vi "sequential on_off - fluigent.vi"() -> ()   [LabVIEW 2018]
doc: "Manually blink and LED attached to a digital output channel of a LINX device by clicking and LED control in LabVIEW."
uses:
  <userlib>/Fluigent/Fluigent MFCS/FluigentMFCS_Full.llb/MFCS_EZ Detect.vi
  <userlib>/Fluigent/Fluigent MFCS/FluigentMFCS_Full.llb/MFCS_EZ Initialization.vi
  <userlib>/Fluigent/Fluigent MFCS/FluigentMFCS_Full.llb/MFCS_EZ Read All Channels Pressure.vi
  <userlib>/Fluigent/Fluigent MFCS/FluigentMFCS_Full.llb/MFCS_EZ Write Channel Pressure.vi
  <userlib>/Fluigent/Fluigent MFCS/FluigentMFCS_Full.llb/MFCS_EZ Close.vi
panel:
  in  "Alpha_8":dbl
  in  "Alpha_7":dbl
  in  "Alpha_6":dbl
  in  "Alpha_5":dbl
  in  "Alpha_4":dbl
  in  "Alpha_3":dbl
  in  "Alpha_2":dbl
  in  "Alpha_1":dbl
  in  "Delay_outlet(ms)":dbl
  in  "Delay_inlet(ms)":dbl
  out "All Channels Pressure":dbl[](array[numeric])
  in  "ch_4_LOW 2":dbl
  in  "ch_3_LOW 2":dbl
  in  "ch_2_LOW 2":dbl
  in  "ch_1_LOW 2":dbl
  in  "ch_4_HIGH 2":dbl
  in  "ch_3_HIGH 2":dbl
  in  "ch_2_HIGH 2":dbl
  in  "ch_1_HIGH 2":dbl
  in  "valve_8_pressure":dbl
  in  "valve_7_pressure":dbl
  in  "valve_6_pressure":dbl
  in  "valve_5_pressure":dbl
  in  "valve_4_pressure":dbl
  in  "valve_3_pressure":dbl
  in  "valve_2_pressure":dbl
  in  "valve_1_pressure":dbl
  in  "ch_4_LOW":dbl
  in  "ch_4_HIGH":dbl
  in  "ch_3_LOW":dbl
  in  "ch_3_HIGH":dbl
  in  "ch_2_LOW":dbl
  in  "ch_2_HIGH":dbl
  in  "ch_1_LOW":dbl
  in  "ch_1_HIGH":dbl
  in  "Chnl_1":bool
  in  "Chnl_2":bool
  in  "Chnl_4":bool
  in  "Chnl_3":bool
  in  "Delay (ms)":dbl
  in  "Mode Selection":enum32{"Manual Control", "Sequential Control"}(radio)
  out "ch_4":bool
  out "ch_3":bool
  out "ch_2":bool
  out "ch_1":bool
  out "id_8":bool
  out "id_7":bool
  out "id_6":bool
  out "id_5":bool
  out "id_4":bool
  out "id_3":bool
  out "id_2":bool
  out "id_1":bool
  in  "stop":bool
  in  "Valve 8":bool
  in  "Valve 7":bool
  in  "Valve 6":bool
  in  "Valve 5":bool
  in  "Valve 4":bool
  in  "Valve 3":bool
  in  "Valve 2":bool
  in  "Valve_1":bool
  # "Manual Control:"
  # "LINX Device Settings"
  # "Sequential Control:"
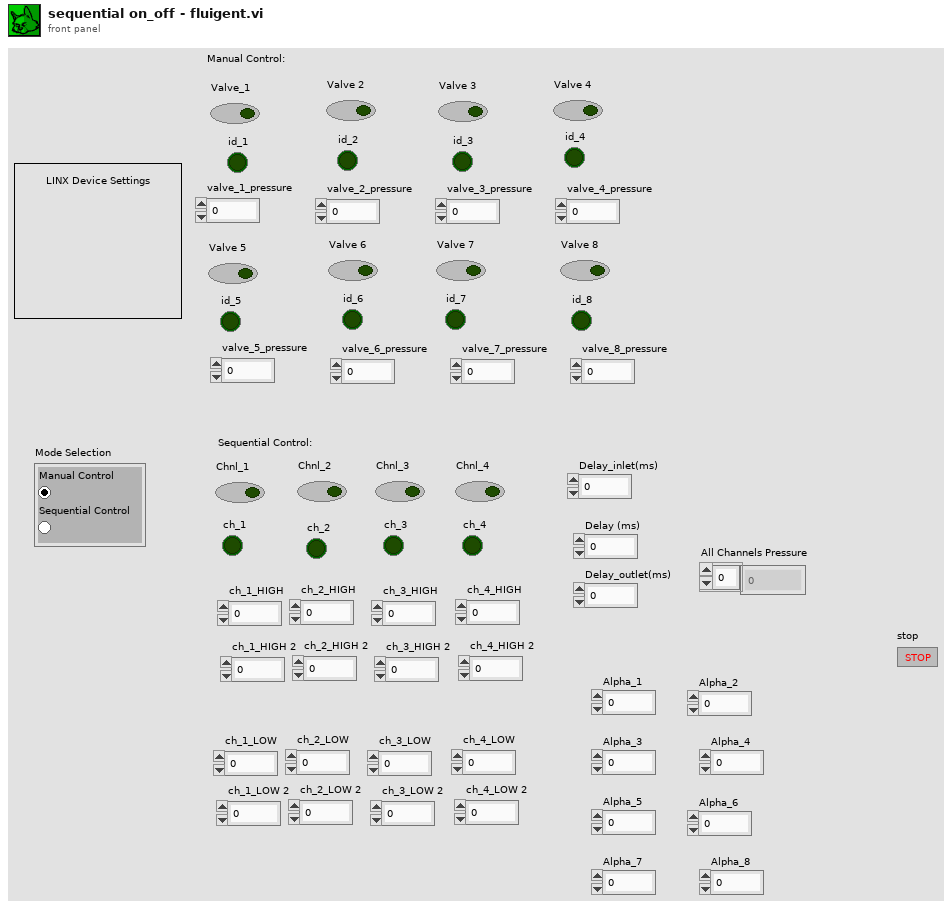
[diagram p1: front panel]
types:
  T1 = typedef "_EZmfcsSN.ctl" = u16
  T2 = typedef "_mfcs_EZ_handle.ctl" = u64
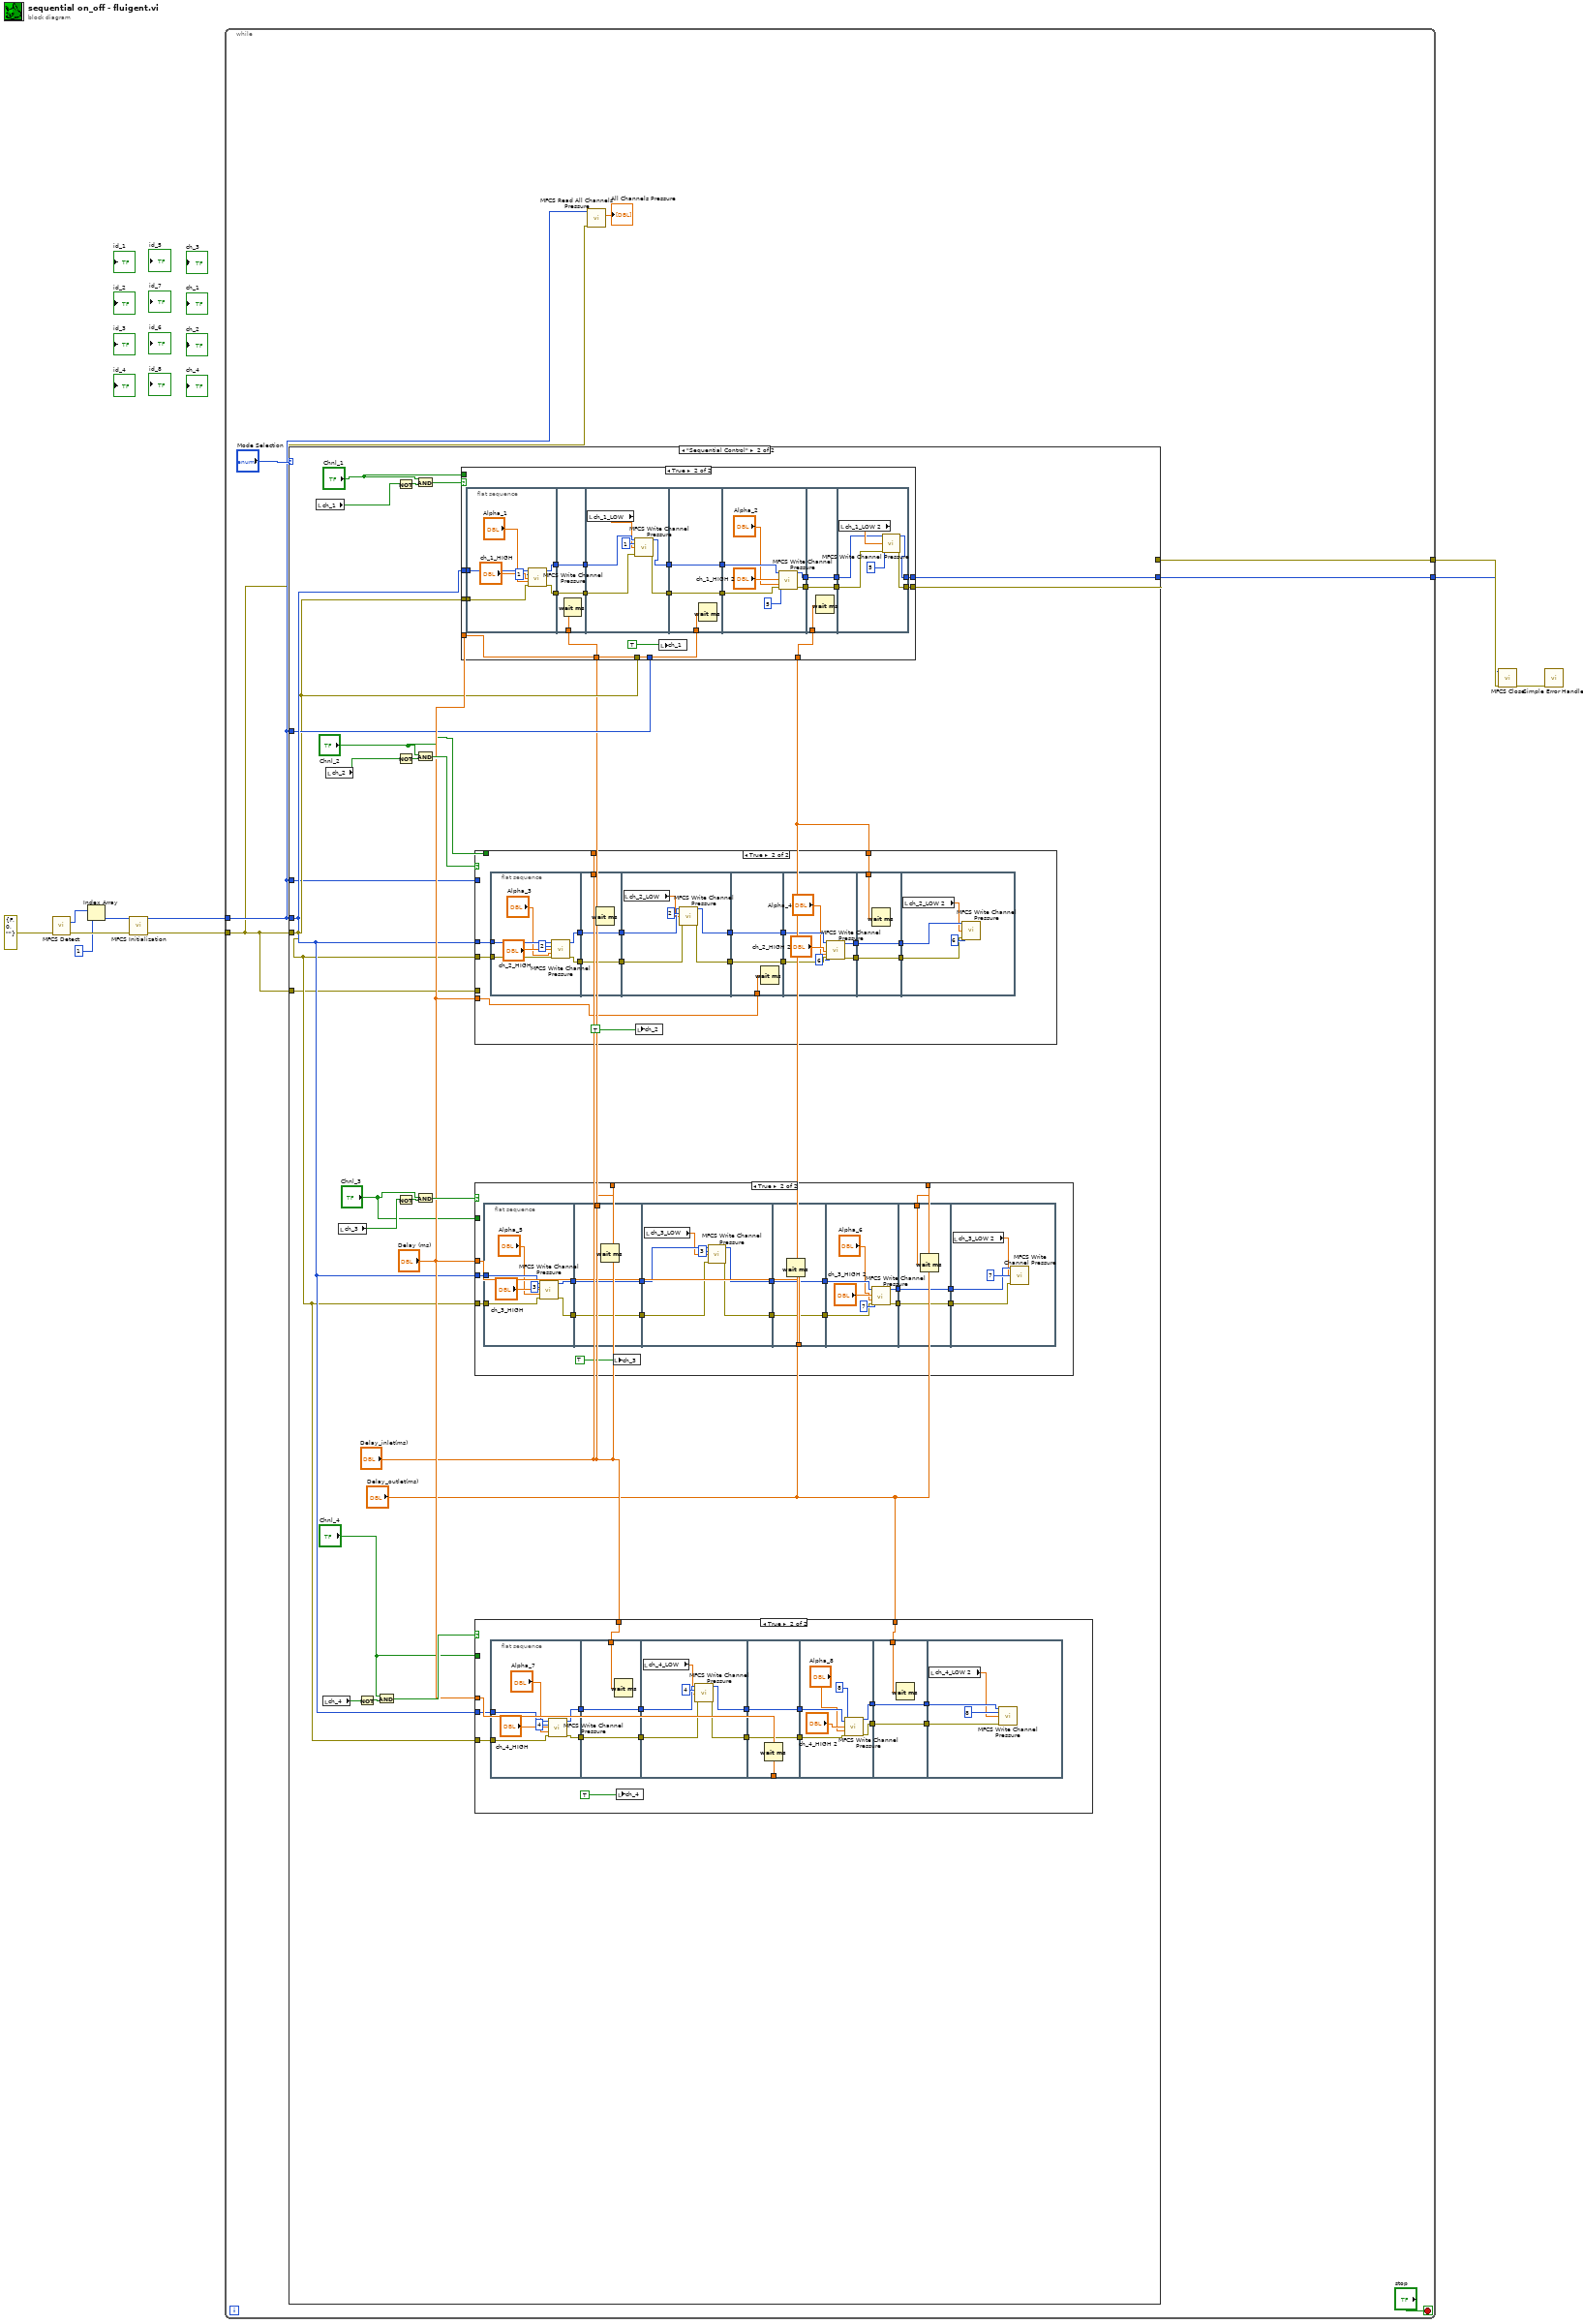
[diagram p0: block diagram]
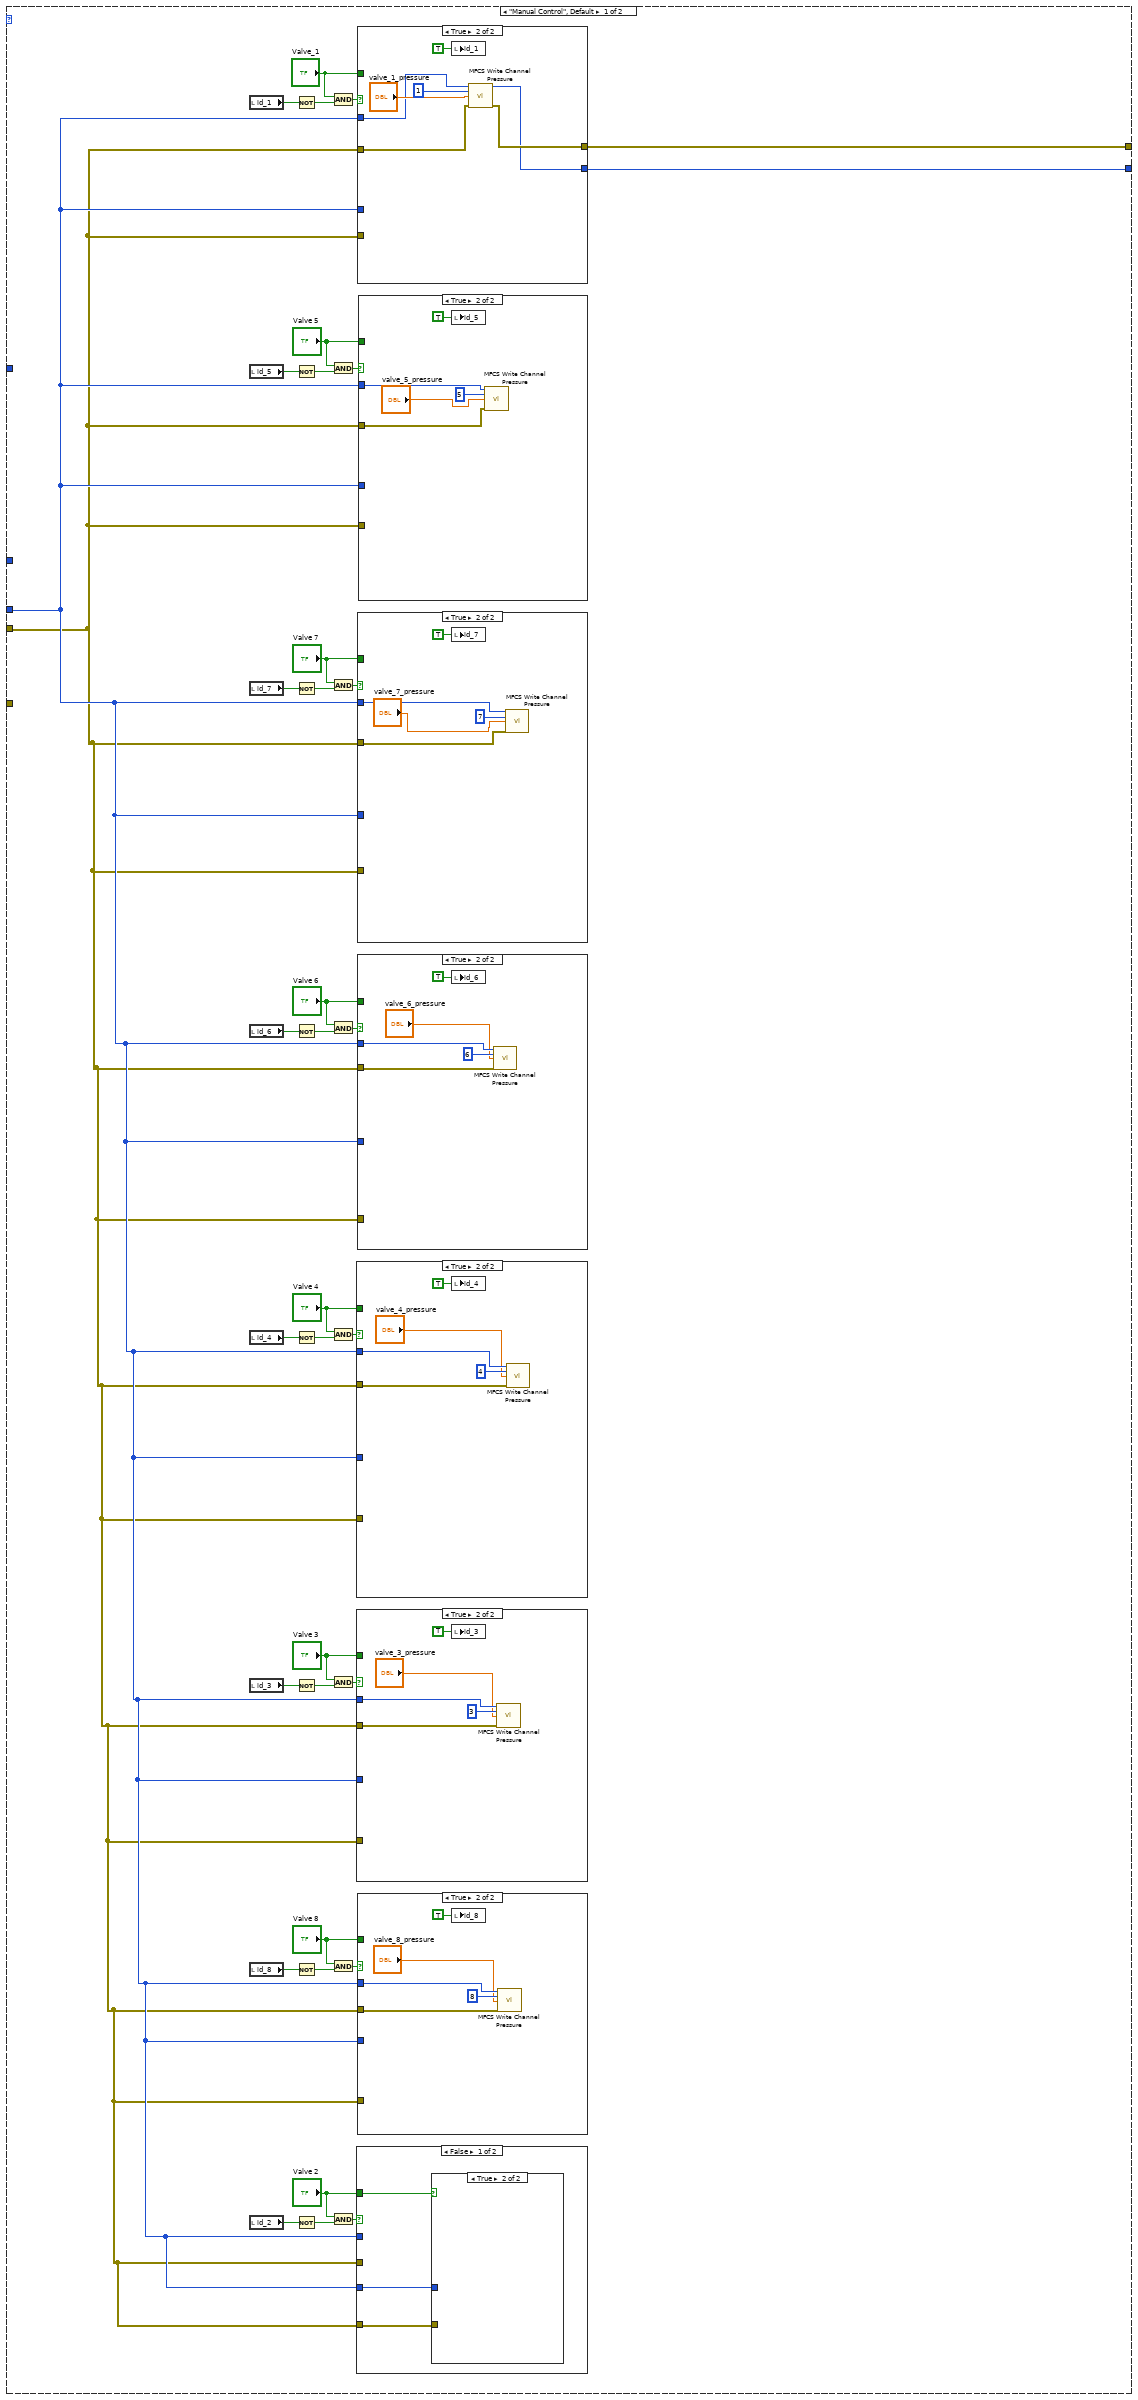
[diagram p2: hidden frame]
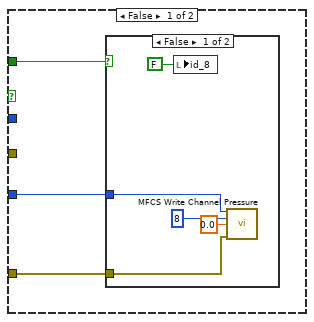
[diagram p3: hidden frame]
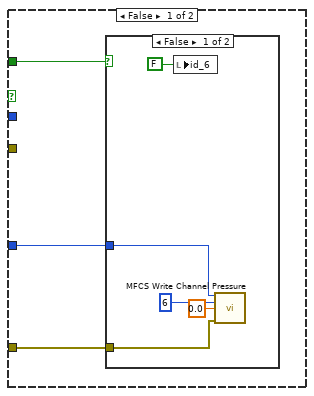
[diagram p5: hidden frame]
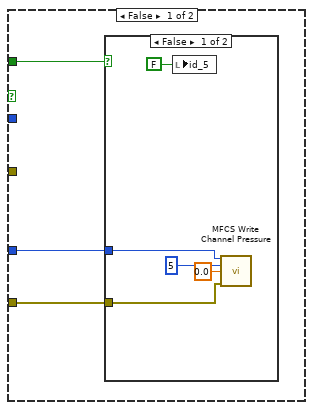
[diagram p7: hidden frame]
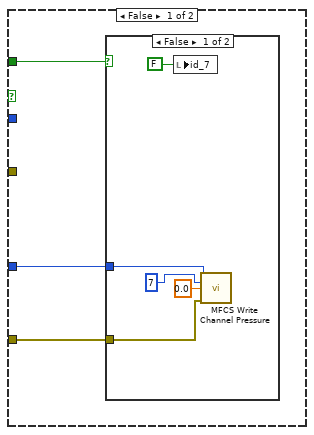
[diagram p9: hidden frame]
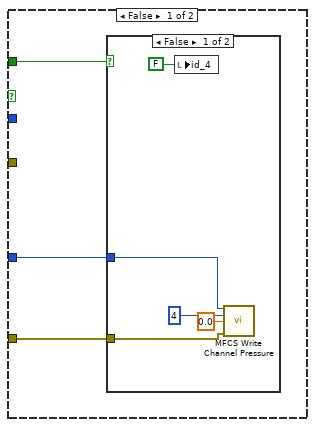
[diagram p11: hidden frame]
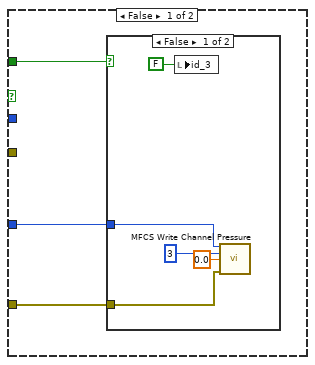
[diagram p13: hidden frame]
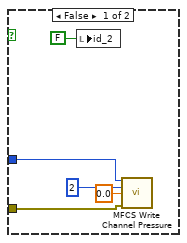
[diagram p15: hidden frame]
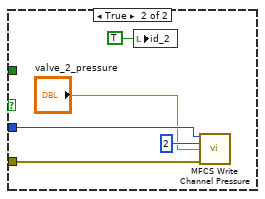
[diagram p16: hidden frame]
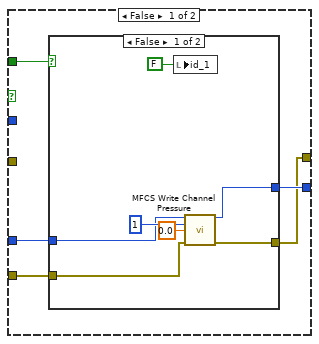
[diagram p17: hidden frame]
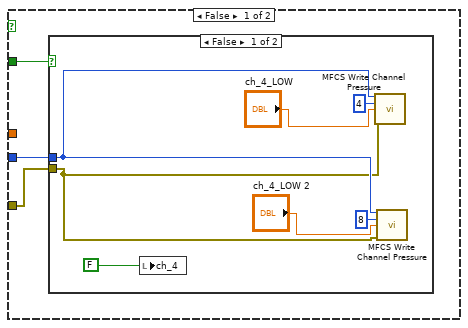
[diagram p19: hidden frame]
diagram:
  n1 = call-poly <userlib>:"MFCS Detect.vi"("error in (no error)"=errorcluster {"status"=FALSE, "code"=0, "source"=""}) -> ("[SN MFCS_EZ]"=w9:T1[], "error out"=w8:errorcluster)  [unwired: 13 in]
  n2 = Index Array(array=w9, index=1) -> (element=w7:T1)
  n3 = call-poly <userlib>:"MFCS Initialization.vi"("SN MFCS_EZ"=w7, "error in (no error)"=w8) -> ("MFCS_EZ_out"=w5:T2, "error out"=w6:errorcluster)  [unwired: 10 in, 2 out]
  n4 = while {
    tunnel: w6 -> [w12]
    tunnel: w5 -> [w13]
    tunnel: [w15] -> w3
    tunnel: [w14] -> w2
    stop <- "stop" stop-if-true
    n5 = case shown="\"Sequential Control\"" "Mode Selection" {
      tunnel: w12 -> [w18 w170]
      tunnel: w13 -> [w19 w172]
      tunnel: [w21 w173] -> w15
      tunnel: [w20 w174] -> w14
      tunnel: w13 -> [_ w171]
      tunnel: w13 -> [_ w169]
      tunnel: w12 -> [_ w168]
      frame "Manual Control", Default {
        n6 = local read "id_1"() -> (w23:bool)
        n7 = local read "id_5"() -> (w36:bool)
        n8 = local read "id_7"() -> (w38:bool)
        n9 = local read "id_6"() -> (w37:bool)
        n10 = local read "id_4"() -> (w35:bool)
        n11 = local read "id_3"() -> (w34:bool)
        n12 = local read "id_8"() -> (w39:bool)
        n13 = local read "id_2"() -> (w27:bool)
        n14 = Not(x=w23) -> (.not. x?=w24:bool)
        n15 = Not(x=w36) -> (.not. x?=w46:bool)
        n16 = Not(x=w38) -> (.not. x?=w42:bool)
        n17 = Not(x=w37) -> (.not. x?=w44:bool)
        n18 = Not(x=w35) -> (.not. x?=w32:bool)
        n19 = Not(x=w34) -> (.not. x?=w29:bool)
        n20 = Not(x=w39) -> (.not. x?=w40:bool)
        n21 = Not(x=w27) -> (.not. x?=w26:bool)
        n22 = And(x="Valve_1", y=w24) -> (x .and. y?=w22:bool)
        n23 = And(x="Valve 5", y=w46) -> (x .and. y?=w47:bool)
        n24 = And(x="Valve 7", y=w42) -> (x .and. y?=w43:bool)
        n25 = And(x="Valve 6", y=w44) -> (x .and. y?=w45:bool)
        n26 = And(x="Valve 4", y=w32) -> (x .and. y?=w33:bool)
        n27 = And(x="Valve 3", y=w29) -> (x .and. y?=w30:bool)
        n28 = And(x="Valve 8", y=w40) -> (x .and. y?=w41:bool)
        n29 = And(x="Valve 2", y=w26) -> (x .and. y?=w25:bool)
        n30 = case shown="True" w33 {
          tunnel: "Valve 4" -> [w108 _]
          tunnel: w19 -> [_ w116]
          tunnel: w18 -> [_ w115]
          tunnel: w19 -> [w107 _]
          tunnel: w18 -> [w106 _]
          frame False {
            n31 = case shown="False" w108 {
              tunnel: w107 -> [w110 _]
              tunnel: w106 -> [w109 _]
              frame False {
                n32 = local write "id_4"(FALSE) -> ()
                n33 = call-poly <userlib>:"MFCS Write Channel Pressure.vi"("MFCS_EZ"=w110, "Channel Number (default=1)"=u8 4, "Pressure (mBar)"=0.0, "error in (no error)"=w109) -> ()  [unwired: 10 in, 2 out]
              }
              frame True {
              }
            }
          }
          frame True {
            n34 = local write "id_4"(TRUE) -> ()
            n35 = call-poly <userlib>:"MFCS Write Channel Pressure.vi"("MFCS_EZ"=w116, "Channel Number (default=1)"=u8 4, "Pressure (mBar)"="valve_4_pressure", "error in (no error)"=w115) -> ()  [unwired: 10 in, 2 out]
          }
        }
        n36 = case shown="True" w30 {
          tunnel: "Valve 3" -> [w121 _]
          tunnel: w19 -> [_ w129]
          tunnel: w18 -> [_ w128]
          tunnel: w19 -> [w120 _]
          tunnel: w18 -> [w119 _]
          frame False {
            n37 = case shown="False" w121 {
              tunnel: w120 -> [w123 _]
              tunnel: w119 -> [w122 _]
              frame False {
                n38 = local write "id_3"(FALSE) -> ()
                n39 = call-poly <userlib>:"MFCS Write Channel Pressure.vi"("MFCS_EZ"=w123, "Channel Number (default=1)"=u8 3, "Pressure (mBar)"=0.0, "error in (no error)"=w122) -> ()  [unwired: 10 in, 2 out]
              }
              frame True {
              }
            }
          }
          frame True {
            n40 = local write "id_3"(TRUE) -> ()
            n41 = call-poly <userlib>:"MFCS Write Channel Pressure.vi"("MFCS_EZ"=w129, "Channel Number (default=1)"=u8 3, "Pressure (mBar)"="valve_3_pressure", "error in (no error)"=w128) -> ()  [unwired: 10 in, 2 out]
          }
        }
        n42 = case shown="False" w25 {
          tunnel: "Valve 2" -> [w134 _]
          tunnel: w19 -> [_ w142]
          tunnel: w18 -> [_ w141]
          tunnel: w19 -> [w133 _]
          tunnel: w18 -> [w132 _]
          frame False {
            n43 = case shown="True" w134 {
              tunnel: w133 -> [w136 _]
              tunnel: w132 -> [w135 _]
              frame False {
                n44 = local write "id_2"(FALSE) -> ()
                n45 = call-poly <userlib>:"MFCS Write Channel Pressure.vi"("MFCS_EZ"=w136, "Channel Number (default=1)"=u8 2, "Pressure (mBar)"=0.0, "error in (no error)"=w135) -> ()  [unwired: 10 in, 2 out]
              }
              frame True {
              }
            }
          }
          frame True {
            n46 = local write "id_2"(TRUE) -> ()
            n47 = call-poly <userlib>:"MFCS Write Channel Pressure.vi"("MFCS_EZ"=w142, "Channel Number (default=1)"=u8 2, "Pressure (mBar)"="valve_2_pressure", "error in (no error)"=w141) -> ()  [unwired: 10 in, 2 out]
          }
        }
        n48 = case shown="True" w22 {
          tunnel: "Valve_1" -> [w149 _]
          tunnel: w18 -> [_ w163]
          tunnel: w19 -> [_ w162]
          tunnel: [w145 w161] -> w21
          tunnel: [w146 w160] -> w20
          tunnel: w19 -> [w148 _]
          tunnel: w18 -> [w147 _]
          frame False {
            n49 = case shown="False" w149 {
              tunnel: w148 -> [w154 w158]
              tunnel: w147 -> [w152 w157]
              tunnel: [w151 w158] -> w146
              tunnel: [w150 w157] -> w145
              frame False {
                n50 = local write "id_1"(FALSE) -> ()
                n51 = call-poly <userlib>:"MFCS Write Channel Pressure.vi"("MFCS_EZ"=w154, "Channel Number (default=1)"=u8 1, "Pressure (mBar)"=0.0, "error in (no error)"=w152) -> ("MFCS_EZ out"=w151:T2, "error out"=w150:errorcluster)  [unwired: 10 in]
              }
              frame True {
              }
            }
          }
          frame True {
            n52 = local write "id_1"(TRUE) -> ()
            n53 = call-poly <userlib>:"MFCS Write Channel Pressure.vi"("MFCS_EZ"=w162, "Channel Number (default=1)"=u8 1, "Pressure (mBar)"="valve_1_pressure", "error in (no error)"=w163) -> ("MFCS_EZ out"=w160:T2, "error out"=w161:errorcluster)  [unwired: 10 in]
          }
        }
        n54 = case shown="True" w43 {
          tunnel: "Valve 7" -> [w95 _]
          tunnel: w18 -> [_ w103]
          tunnel: w19 -> [_ w102]
          tunnel: w19 -> [w94 _]
          tunnel: w18 -> [w93 _]
          frame False {
            n55 = case shown="False" w95 {
              tunnel: w94 -> [w97 _]
              tunnel: w93 -> [w96 _]
              frame False {
                n56 = local write "id_7"(FALSE) -> ()
                n57 = call-poly <userlib>:"MFCS Write Channel Pressure.vi"("MFCS_EZ"=w97, "Channel Number (default=1)"=u8 7, "Pressure (mBar)"=0.0, "error in (no error)"=w96) -> ()  [unwired: 10 in, 2 out]
              }
              frame True {
              }
            }
          }
          frame True {
            n58 = local write "id_7"(TRUE) -> ()
            n59 = call-poly <userlib>:"MFCS Write Channel Pressure.vi"("MFCS_EZ"=w102, "Channel Number (default=1)"=u8 7, "Pressure (mBar)"="valve_7_pressure", "error in (no error)"=w103) -> ()  [unwired: 10 in, 2 out]
          }
        }
        n60 = case shown="True" w45 {
          tunnel: "Valve 6" -> [w69 _]
          tunnel: w19 -> [_ w77]
          tunnel: w18 -> [_ w76]
          tunnel: w19 -> [w68 _]
          tunnel: w18 -> [w67 _]
          frame False {
            n61 = case shown="False" w69 {
              tunnel: w68 -> [w71 _]
              tunnel: w67 -> [w70 _]
              frame False {
                n62 = local write "id_6"(FALSE) -> ()
                n63 = call-poly <userlib>:"MFCS Write Channel Pressure.vi"("MFCS_EZ"=w71, "Channel Number (default=1)"=u8 6, "Pressure (mBar)"=0.0, "error in (no error)"=w70) -> ()  [unwired: 10 in, 2 out]
              }
              frame True {
              }
            }
          }
          frame True {
            n64 = local write "id_6"(TRUE) -> ()
            n65 = call-poly <userlib>:"MFCS Write Channel Pressure.vi"("MFCS_EZ"=w77, "Channel Number (default=1)"=u8 6, "Pressure (mBar)"="valve_6_pressure", "error in (no error)"=w76) -> ()  [unwired: 10 in, 2 out]
          }
        }
        n66 = case shown="True" w41 {
          tunnel: "Valve 8" -> [w56 _]
          tunnel: w19 -> [_ w64]
          tunnel: w18 -> [_ w63]
          tunnel: w19 -> [w55 _]
          tunnel: w18 -> [w54 _]
          frame False {
            n67 = case shown="False" w56 {
              tunnel: w55 -> [w58 _]
              tunnel: w54 -> [w57 _]
              frame False {
                n68 = local write "id_8"(FALSE) -> ()
                n69 = call-poly <userlib>:"MFCS Write Channel Pressure.vi"("MFCS_EZ"=w58, "Channel Number (default=1)"=u8 8, "Pressure (mBar)"=0.0, "error in (no error)"=w57) -> ()  [unwired: 10 in, 2 out]
              }
              frame True {
              }
            }
          }
          frame True {
            n70 = local write "id_8"(TRUE) -> ()
            n71 = call-poly <userlib>:"MFCS Write Channel Pressure.vi"("MFCS_EZ"=w64, "Channel Number (default=1)"=u8 8, "Pressure (mBar)"="valve_8_pressure", "error in (no error)"=w63) -> ()  [unwired: 10 in, 2 out]
          }
        }
        n72 = case shown="True" w47 {
          tunnel: "Valve 5" -> [w82 _]
          tunnel: w19 -> [_ w91]
          tunnel: w18 -> [_ w90]
          tunnel: w19 -> [w81 _]
          tunnel: w18 -> [w80 _]
          frame False {
            n73 = case shown="False" w82 {
              tunnel: w81 -> [w84 _]
              tunnel: w80 -> [w83 _]
              frame False {
                n74 = local write "id_5"(FALSE) -> ()
                n75 = call-poly <userlib>:"MFCS Write Channel Pressure.vi"("MFCS_EZ"=w84, "Channel Number (default=1)"=u8 5, "Pressure (mBar)"=0.0, "error in (no error)"=w83) -> ()  [unwired: 10 in, 2 out]
              }
              frame True {
              }
            }
          }
          frame True {
            n76 = local write "id_5"(TRUE) -> ()
            n77 = call-poly <userlib>:"MFCS Write Channel Pressure.vi"("MFCS_EZ"=w91, "Channel Number (default=1)"=u8 5, "Pressure (mBar)"="valve_5_pressure", "error in (no error)"=w90) -> ()  [unwired: 10 in, 2 out]
          }
        }
      }
      frame "Sequential Control" {
        n78 = local read "ch_1"() -> (w182:bool)
        n79 = local read "ch_4"() -> (w176:bool)
        n80 = local read "ch_2"() -> (w179:bool)
        n81 = local read "ch_3"() -> (w178:bool)
        n82 = Not(x=w176) -> (.not. x?=w185:bool)
        n83 = And(x="Chnl_4", y=w185) -> (x .and. y?=w184:bool)
        n84 = Not(x=w182) -> (.not. x?=w191:bool)
        n85 = Not(x=w179) -> (.not. x?=w189:bool)
        n86 = Not(x=w178) -> (.not. x?=w187:bool)
        n87 = And(x="Chnl_1", y=w191) -> (x .and. y?=w190:bool)
        n88 = And(x="Chnl_2", y=w189) -> (x .and. y?=w188:bool)
        n89 = And(x="Chnl_3", y=w187) -> (x .and. y?=w186:bool)
        n90 = case shown="True" w190 {
          tunnel: "Delay (ms)" -> [_ w411]
          tunnel: "Chnl_1" -> [w380 _]
          tunnel: w172 -> [_ w409]
          tunnel: w170 -> [w375 w408]
          tunnel: [w377 w405] -> w174
          tunnel: [w376 w404] -> w173
          tunnel: w171 -> [w379 _]
          tunnel: w170 -> [w378 _]
          tunnel: "Delay_inlet(ms)" -> [_ w393]
          tunnel: "Delay_outlet(ms)" -> [_ w392]
          frame False {
            n91 = case shown="False" w380 {
              tunnel: w379 -> [w388 w391]
              tunnel: w378 -> [w387 _]
              tunnel: [w382 w391] -> w377
              tunnel: [w381 w390] -> w376
              tunnel: w375 -> [_ w390]
              frame False {
                n92 = local write "ch_1"(FALSE) -> ()
                n93 = call-poly <userlib>:"MFCS Write Channel Pressure.vi"("MFCS_EZ"=w388, "Channel Number (default=1)"=u8 1, "Pressure (mBar)"="ch_1_LOW", "error in (no error)"=w387) -> ()  [unwired: 10 in, 2 out]
                n94 = call-poly <userlib>:"MFCS Write Channel Pressure.vi"("MFCS_EZ"=w388, "Channel Number (default=1)"=u8 5, "Pressure (mBar)"="ch_1_LOW 2", "error in (no error)"=w387) -> ("MFCS_EZ out"=w382:T2, "error out"=w381:errorcluster)  [unwired: 10 in]
              }
              frame True {
              }
            }
          }
          frame True {
            n95 = flat-sequence {
              tunnel: w409 -> [w418]
              tunnel: w408 -> [w417]
              tunnel: [w414] -> w403
              tunnel: [w413] -> w402
              tunnel: w403 -> [w421]
              tunnel: [w421] -> w401
              tunnel: w402 -> [w420]
              tunnel: [w420] -> w399
              tunnel: w393 -> [w419]
              tunnel: w401 -> [w423]
              tunnel: [w422] -> w400
              tunnel: w399 -> [w426]
              tunnel: [w425] -> w398
              tunnel: w411 -> [w430]
              tunnel: [w429] -> w407
              tunnel: w400 -> [w429]
              tunnel: [w428] -> w406
              tunnel: w398 -> [w428]
              tunnel: w407 -> [w436]
              tunnel: w406 -> [w435]
              tunnel: [w433] -> w397
              tunnel: [w432] -> w396
              tunnel: w397 -> [w440]
              tunnel: w396 -> [w439]
              tunnel: [w440] -> w395
              tunnel: [w439] -> w394
              tunnel: w392 -> [w438]
              tunnel: [w441] -> w404
              tunnel: [w443] -> w405
              tunnel: w395 -> [w444]
              tunnel: w394 -> [w442]
              frame #0 {
                n96 = call-poly <userlib>:"MFCS Write Channel Pressure.vi"("MFCS_EZ"=w418, "Channel Number (default=1)"=u8 1, "Pressure (mBar)"="ch_1_HIGH", "Alpha (default=5)"="Alpha_1", "error in (no error)"=w417) -> ("MFCS_EZ out"=w413:T2, "error out"=w414:errorcluster)  [unwired: 9 in]
              }
              frame #1 {
                n97 = Wait (ms)(milliseconds to wait=w419) -> ()  [unwired: 1 out]
              }
              frame #2 {
                n98 = local read "ch_1_LOW"() -> (w424:dbl)
                n99 = call-poly <userlib>:"MFCS Write Channel Pressure.vi"("MFCS_EZ"=w426, "Channel Number (default=1)"=u8 1, "Pressure (mBar)"=w424, "error in (no error)"=w423) -> ("MFCS_EZ out"=w425:T2, "error out"=w422:errorcluster)  [unwired: 10 in]
              }
              frame #3 {
                n100 = Wait (ms)(milliseconds to wait=w430) -> ()  [unwired: 1 out]
              }
              frame #4 {
                n101 = call-poly <userlib>:"MFCS Write Channel Pressure.vi"("MFCS_EZ"=w435, "Channel Number (default=1)"=u8 5, "Pressure (mBar)"="ch_1_HIGH 2", "Alpha (default=5)"="Alpha_2", "error in (no error)"=w436) -> ("MFCS_EZ out"=w433:T2, "error out"=w432:errorcluster)  [unwired: 9 in]
              }
              frame #5 {
                n102 = Wait (ms)(milliseconds to wait=w438) -> ()  [unwired: 1 out]
              }
              frame #6 {
                n103 = local read "ch_1_LOW 2"() -> (w445:dbl)
                n104 = call-poly <userlib>:"MFCS Write Channel Pressure.vi"("MFCS_EZ"=w444, "Channel Number (default=1)"=u8 5, "Pressure (mBar)"=w445, "error in (no error)"=w442) -> ("MFCS_EZ out"=w443:T2, "error out"=w441:errorcluster)  [unwired: 10 in]
              }
            }
            n105 = local write "ch_1"(TRUE) -> ()
          }
        }
        n106 = case shown="True" w188 {
          tunnel: "Delay (ms)" -> [_ w341]
          tunnel: "Chnl_2" -> [w316 _]
          tunnel: w172 -> [_ w339]
          tunnel: w170 -> [_ w338]
          tunnel: w169 -> [w315 _]
          tunnel: w168 -> [w314 _]
          tunnel: "Delay_inlet(ms)" -> [_ w325]
          tunnel: "Delay_outlet(ms)" -> [_ w324]
          frame False {
            n107 = case shown="False" w316 {
              tunnel: w315 -> [w318 _]
              tunnel: w314 -> [w317 _]
              frame False {
                n108 = local write "ch_2"(FALSE) -> ()
                n109 = call-poly <userlib>:"MFCS Write Channel Pressure.vi"("MFCS_EZ"=w318, "Channel Number (default=1)"=u8 2, "Pressure (mBar)"="ch_2_LOW", "error in (no error)"=w317) -> ()  [unwired: 10 in, 2 out]
                n110 = call-poly <userlib>:"MFCS Write Channel Pressure.vi"("MFCS_EZ"=w318, "Channel Number (default=1)"=u8 6, "Pressure (mBar)"="ch_2_LOW 2", "error in (no error)"=w317) -> ()  [unwired: 10 in, 2 out]
              }
              frame True {
              }
            }
          }
          frame True {
            n111 = flat-sequence {
              tunnel: w339 -> [w348]
              tunnel: w338 -> [w347]
              tunnel: [w346] -> w335
              tunnel: [w345] -> w334
              tunnel: w335 -> [w351]
              tunnel: [w351] -> w333
              tunnel: w334 -> [w350]
              tunnel: [w350] -> w331
              tunnel: w325 -> [w349]
              tunnel: w333 -> [w356]
              tunnel: [w355] -> w332
              tunnel: w331 -> [w354]
              tunnel: [w353] -> w330
              tunnel: w341 -> [w360]
              tunnel: [w359] -> w337
              tunnel: w332 -> [w359]
              tunnel: [w358] -> w336
              tunnel: w330 -> [w358]
              tunnel: w337 -> [w367]
              tunnel: w336 -> [w366]
              tunnel: [w363] -> w328
              tunnel: [w362] -> w326
              tunnel: [w370] -> w329
              tunnel: w328 -> [w370]
              tunnel: [w369] -> w327
              tunnel: w326 -> [w369]
              tunnel: w324 -> [w368]
              tunnel: w329 -> [w373]
              tunnel: w327 -> [w372]
              frame #0 {
                n112 = call-poly <userlib>:"MFCS Write Channel Pressure.vi"("MFCS_EZ"=w348, "Channel Number (default=1)"=u8 2, "Pressure (mBar)"="ch_2_HIGH", "Alpha (default=5)"="Alpha_3", "error in (no error)"=w347) -> ("MFCS_EZ out"=w346:T2, "error out"=w345:errorcluster)  [unwired: 9 in]
              }
              frame #1 {
                n113 = Wait (ms)(milliseconds to wait=w349) -> ()  [unwired: 1 out]
              }
              frame #2 {
                n114 = local read "ch_2_LOW"() -> (w352:dbl)
                n115 = call-poly <userlib>:"MFCS Write Channel Pressure.vi"("MFCS_EZ"=w356, "Channel Number (default=1)"=u8 2, "Pressure (mBar)"=w352, "error in (no error)"=w354) -> ("MFCS_EZ out"=w355:T2, "error out"=w353:errorcluster)  [unwired: 10 in]
              }
              frame #3 {
                n116 = Wait (ms)(milliseconds to wait=w360) -> ()  [unwired: 1 out]
              }
              frame #4 {
                n117 = call-poly <userlib>:"MFCS Write Channel Pressure.vi"("MFCS_EZ"=w367, "Channel Number (default=1)"=u8 6, "Pressure (mBar)"="ch_2_HIGH 2", "Alpha (default=5)"="Alpha_4", "error in (no error)"=w366) -> ("MFCS_EZ out"=w363:T2, "error out"=w362:errorcluster)  [unwired: 9 in]
              }
              frame #5 {
                n118 = Wait (ms)(milliseconds to wait=w368) -> ()  [unwired: 1 out]
              }
              frame #6 {
                n119 = local read "ch_2_LOW 2"() -> (w371:dbl)
                n120 = call-poly <userlib>:"MFCS Write Channel Pressure.vi"("MFCS_EZ"=w373, "Channel Number (default=1)"=u8 6, "Pressure (mBar)"=w371, "error in (no error)"=w372) -> ()  [unwired: 10 in, 2 out]
              }
            }
            n121 = local write "ch_2"(TRUE) -> ()
          }
        }
        n122 = case shown="True" w186 {
          tunnel: "Delay (ms)" -> [_ w280]
          tunnel: "Chnl_3" -> [w255 _]
          tunnel: w172 -> [w254 w276]
          tunnel: w170 -> [w253 w275]
          tunnel: "Delay_inlet(ms)" -> [_ w268]
          tunnel: "Delay_outlet(ms)" -> [_ w267]
          frame False {
            n123 = case shown="False" w255 {
              tunnel: w254 -> [w256 _]
              tunnel: w253 -> [w261 _]
              frame False {
                n124 = local write "ch_3"(FALSE) -> ()
                n125 = call-poly <userlib>:"MFCS Write Channel Pressure.vi"("MFCS_EZ"=w256, "Channel Number (default=1)"=u8 3, "Pressure (mBar)"="ch_3_LOW", "error in (no error)"=w261) -> ()  [unwired: 10 in, 2 out]
                n126 = call-poly <userlib>:"MFCS Write Channel Pressure.vi"("MFCS_EZ"=w256, "Channel Number (default=1)"=u8 7, "Pressure (mBar)"="ch_3_LOW 2", "error in (no error)"=w261) -> ()  [unwired: 10 in, 2 out]
              }
              frame True {
              }
            }
          }
          frame True {
            n127 = flat-sequence {
              tunnel: [w285] -> w274
              tunnel: [w284] -> w273
              tunnel: w276 -> [w283]
              tunnel: w275 -> [w282]
              tunnel: w274 -> [w290]
              tunnel: [w290] -> w272
              tunnel: w273 -> [w289]
              tunnel: [w289] -> w270
              tunnel: w268 -> [w288]
              tunnel: w272 -> [w295]
              tunnel: [w294] -> w271
              tunnel: w270 -> [w293]
              tunnel: [w292] -> w269
              tunnel: w280 -> [w299]
              tunnel: [w298] -> w278
              tunnel: w271 -> [w298]
              tunnel: [w297] -> w277
              tunnel: w269 -> [w297]
              tunnel: w278 -> [w304]
              tunnel: w277 -> [w303]
              tunnel: [w302] -> w265
              tunnel: [w301] -> w263
              tunnel: w267 -> [w309]
              tunnel: [w308] -> w266
              tunnel: w265 -> [w308]
              tunnel: [w307] -> w264
              tunnel: w263 -> [w307]
              tunnel: w266 -> [w312]
              tunnel: w264 -> [w311]
              frame #0 {
                n128 = call-poly <userlib>:"MFCS Write Channel Pressure.vi"("MFCS_EZ"=w283, "Channel Number (default=1)"=u8 3, "Pressure (mBar)"="ch_3_HIGH", "Alpha (default=5)"="Alpha_5", "error in (no error)"=w282) -> ("MFCS_EZ out"=w285:T2, "error out"=w284:errorcluster)  [unwired: 9 in]
              }
              frame #1 {
                n129 = Wait (ms)(milliseconds to wait=w288) -> ()  [unwired: 1 out]
              }
              frame #2 {
                n130 = local read "ch_3_LOW"() -> (w291:dbl)
                n131 = call-poly <userlib>:"MFCS Write Channel Pressure.vi"("MFCS_EZ"=w295, "Channel Number (default=1)"=u8 3, "Pressure (mBar)"=w291, "error in (no error)"=w293) -> ("MFCS_EZ out"=w294:T2, "error out"=w292:errorcluster)  [unwired: 10 in]
              }
              frame #3 {
                n132 = Wait (ms)(milliseconds to wait=w299) -> ()  [unwired: 1 out]
              }
              frame #4 {
                n133 = call-poly <userlib>:"MFCS Write Channel Pressure.vi"("MFCS_EZ"=w304, "Channel Number (default=1)"=u8 7, "Pressure (mBar)"="ch_3_HIGH 2", "Alpha (default=5)"="Alpha_6", "error in (no error)"=w303) -> ("MFCS_EZ out"=w302:T2, "error out"=w301:errorcluster)  [unwired: 9 in]
              }
              frame #5 {
                n134 = Wait (ms)(milliseconds to wait=w309) -> ()  [unwired: 1 out]
              }
              frame #6 {
                n135 = local read "ch_3_LOW 2"() -> (w310:dbl)
                n136 = call-poly <userlib>:"MFCS Write Channel Pressure.vi"("MFCS_EZ"=w312, "Channel Number (default=1)"=u8 7, "Pressure (mBar)"=w310, "error in (no error)"=w311) -> ()  [unwired: 10 in, 2 out]
              }
            }
            n137 = local write "ch_3"(TRUE) -> ()
          }
        }
        n138 = case shown="True" w184 {
          tunnel: "Delay (ms)" -> [_ w219]
          tunnel: "Chnl_4" -> [w194 _]
          tunnel: w172 -> [w193 w215]
          tunnel: w170 -> [w192 w214]
          tunnel: "Delay_inlet(ms)" -> [_ w207]
          tunnel: "Delay_outlet(ms)" -> [_ w206]
          frame False {
            n139 = case shown="False" w194 {
              tunnel: w193 -> [w196 _]
              tunnel: w192 -> [w195 _]
              frame False {
                n140 = local write "ch_4"(FALSE) -> ()
                n141 = call-poly <userlib>:"MFCS Write Channel Pressure.vi"("MFCS_EZ"=w196, "Channel Number (default=1)"=u8 4, "Pressure (mBar)"="ch_4_LOW", "error in (no error)"=w195) -> ()  [unwired: 10 in, 2 out]
                n142 = call-poly <userlib>:"MFCS Write Channel Pressure.vi"("MFCS_EZ"=w196, "Channel Number (default=1)"=u8 8, "Pressure (mBar)"="ch_4_LOW 2", "error in (no error)"=w195) -> ()  [unwired: 10 in, 2 out]
              }
              frame True {
              }
            }
          }
          frame True {
            n143 = flat-sequence {
              tunnel: [w225] -> w213
              tunnel: [w224] -> w212
              tunnel: w215 -> [w223]
              tunnel: w214 -> [w222]
              tunnel: w213 -> [w229]
              tunnel: [w229] -> w211
              tunnel: w212 -> [w228]
              tunnel: [w228] -> w209
              tunnel: w207 -> [w227]
              tunnel: w211 -> [w234]
              tunnel: [w233] -> w210
              tunnel: w209 -> [w232]
              tunnel: [w231] -> w208
              tunnel: w219 -> [w238]
              tunnel: [w237] -> w217
              tunnel: w210 -> [w237]
              tunnel: [w236] -> w216
              tunnel: w208 -> [w236]
              tunnel: w217 -> [w244]
              tunnel: w216 -> [w243]
              tunnel: [w241] -> w204
              tunnel: [w240] -> w202
              tunnel: w206 -> [w248]
              tunnel: [w247] -> w205
              tunnel: w204 -> [w247]
              tunnel: [w246] -> w203
              tunnel: w202 -> [w246]
              tunnel: w205 -> [w251]
              tunnel: w203 -> [w250]
              frame #0 {
                n144 = call-poly <userlib>:"MFCS Write Channel Pressure.vi"("MFCS_EZ"=w223, "Channel Number (default=1)"=u8 4, "Pressure (mBar)"="ch_4_HIGH", "Alpha (default=5)"="Alpha_7", "error in (no error)"=w222) -> ("MFCS_EZ out"=w225:T2, "error out"=w224:errorcluster)  [unwired: 9 in]
              }
              frame #1 {
                n145 = Wait (ms)(milliseconds to wait=w227) -> ()  [unwired: 1 out]
              }
              frame #2 {
                n146 = local read "ch_4_LOW"() -> (w230:dbl)
                n147 = call-poly <userlib>:"MFCS Write Channel Pressure.vi"("MFCS_EZ"=w234, "Channel Number (default=1)"=u8 4, "Pressure (mBar)"=w230, "error in (no error)"=w232) -> ("MFCS_EZ out"=w233:T2, "error out"=w231:errorcluster)  [unwired: 10 in]
              }
              frame #3 {
                n148 = Wait (ms)(milliseconds to wait=w238) -> ()  [unwired: 1 out]
              }
              frame #4 {
                n149 = call-poly <userlib>:"MFCS Write Channel Pressure.vi"("MFCS_EZ"=w244, "Channel Number (default=1)"=u8 8, "Pressure (mBar)"="ch_4_HIGH 2", "Alpha (default=5)"="Alpha_8", "error in (no error)"=w243) -> ("MFCS_EZ out"=w241:T2, "error out"=w240:errorcluster)  [unwired: 9 in]
              }
              frame #5 {
                n150 = Wait (ms)(milliseconds to wait=w248) -> ()  [unwired: 1 out]
              }
              frame #6 {
                n151 = local read "ch_4_LOW 2"() -> (w249:dbl)
                n152 = call-poly <userlib>:"MFCS Write Channel Pressure.vi"("MFCS_EZ"=w251, "Channel Number (default=1)"=u8 8, "Pressure (mBar)"=w249, "error in (no error)"=w250) -> ()  [unwired: 10 in, 2 out]
              }
            }
            n153 = local write "ch_4"(TRUE) -> ()
          }
        }
      }
    }
    n154 = call-poly <userlib>:"MFCS Read All Channels Pressure.vi"("MFCS_EZ"=w13, "error in (no error)"=w12) -> ("All Channels Pressure"=→"All Channels Pressure":dbl[])  [unwired: 11 in, 2 out]
  }
  n155 = call-poly <userlib>:"MFCS Close.vi"("MFCS_EZ"=w2, "error in (no error)"=w3) -> ("error out"=w4:errorcluster)  [unwired: 13 in]
  n156 = call <vilib>:"Simple Error Handler.vi"("error in (no error)"=w4) -> ()  [unwired: 4 in, 5 out]
